vi "Read TestStatus.vi"(11 "Logger in":refnum<class "Logger.lvclass">) -> (2 "TestStatus":T1 {"activeProfileStep" min=1; "activeCycle" min=1}, 3 "Logger out":refnum<class "Logger.lvclass">)   [LabVIEW 2013, in "Logger.lvclass"]
uses:
  Logger.lvclass
  Typedefs/TestStatus.ctl
  Logger.lvclass/Logger.ctl
  Typedefs/M2AADTTypedefs.lvlib
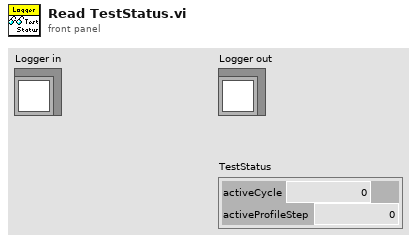
[diagram p1: front panel]
types:
  T1 = typedef "M2AADTTypedefs.lvlib/TestStatus.ctl" = cluster{"activeCycle":u32, "activeProfileStep":u32}
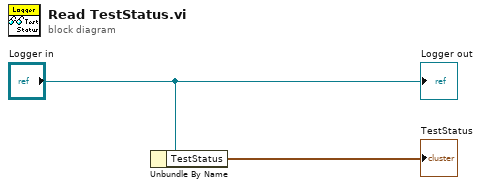
[diagram p0: block diagram]
diagram:
  n1 = Unbundle By Name("Logger in") -> ("TestStatus"=→"TestStatus":T1)
  "Logger out" <- "Logger in"
